vi "Main.vi"() -> ()   [LabVIEW 2012]
doc: "该连续测量范例项目在队列消息处理器模板的基础上实现。\n\n事件处理循环负责按用户界面操作生成对应的消息。\n\n消息处理循环负责对事件处理循环或其他消息生成的消息进行处理。其中还包括用于采集和记录消息处理循环的子VI，以及用于更新图表的循环。"
uses:
  Settings/Settings.ctl
  Acquisition/Hardware Configuration.ctl
  Acquisition/Signal Type.ctl
  Logging/Logging Configuration.ctl
  controls/UI Data.ctl
  Acquisition/Acquisition.lvlib
  Logging/Logging.lvlib
  Settings/Settings.lvlib
  support/User Event - Stop/User Event - Stop.lvlib
  support/Message Queue/Message Queue.lvlib
  Testing/Testing.lvlib
panel:
  out "数据":waveform(dbl)[](graph)
  in  "空白按钮 6":bool
  in  "?":bool
  in  "风机测试":bool
  in  "滚刷测试":bool
  in  "边刷测试":bool
  in  "行走轮测试":bool
  in  "设置":bool
  in  "整机测试开始":bool
  in  "停止":bool
  out "状态":string
  in  "紧急停止按钮":bool
  in  "退出":bool
  # "连续测量数据记录器"
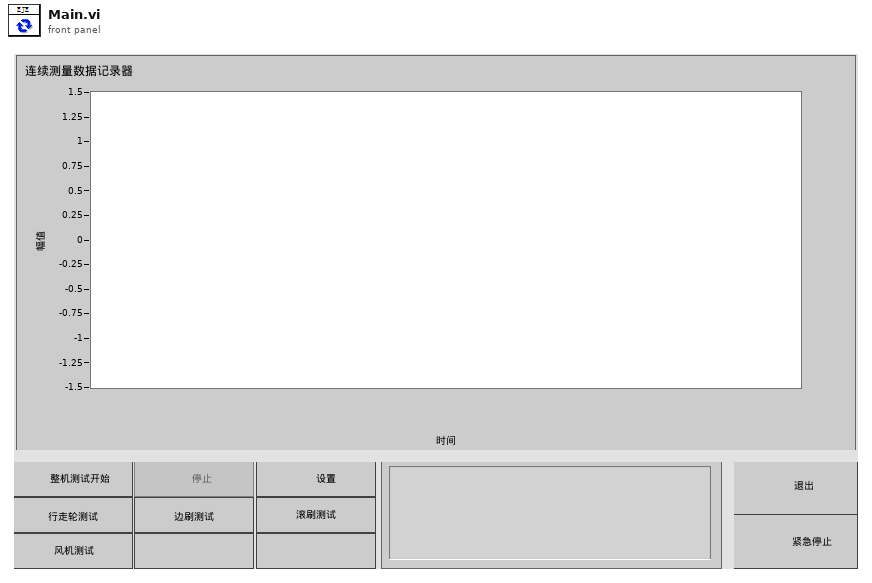
[diagram p1: front panel]
types:
  T1 = typedef "UI Data.ctl" = cluster{"开始引用":refnum<vi>, "停止引用":refnum<vi>, "设置引用":refnum<vi>, "退出引用":refnum<vi>, "状态引用":refnum<vi>, "数据引用":refnum<vi>}
  T2 = typedef "Settings.lvlib/Settings.ctl" = cluster{"硬件配置":T3, "记录配置":T5}
  T3 = typedef "Acquisition.lvlib/Hardware Configuration.ctl" = cluster{"硬件引用句柄<替换此项>":string, "信号类型<替换该项>":T4, "VISA资源名称":refnum<visa-resource-name>}
  T4 = typedef "Acquisition.lvlib/Signal Type.ctl" = enum16{"Sine Wave", "Square with Noise"}
  T5 = typedef "Logging.lvlib/Logging Configuration.ctl" = cluster{"记录文件基路径":path, "TDMS文件引用":refnum<k34>}
  T6 = typedef "Message Queue.lvlib/All Message Queues.ctl" = cluster{"UI":refnum<queue>, "采集":refnum<queue>, "记录":refnum<queue>}
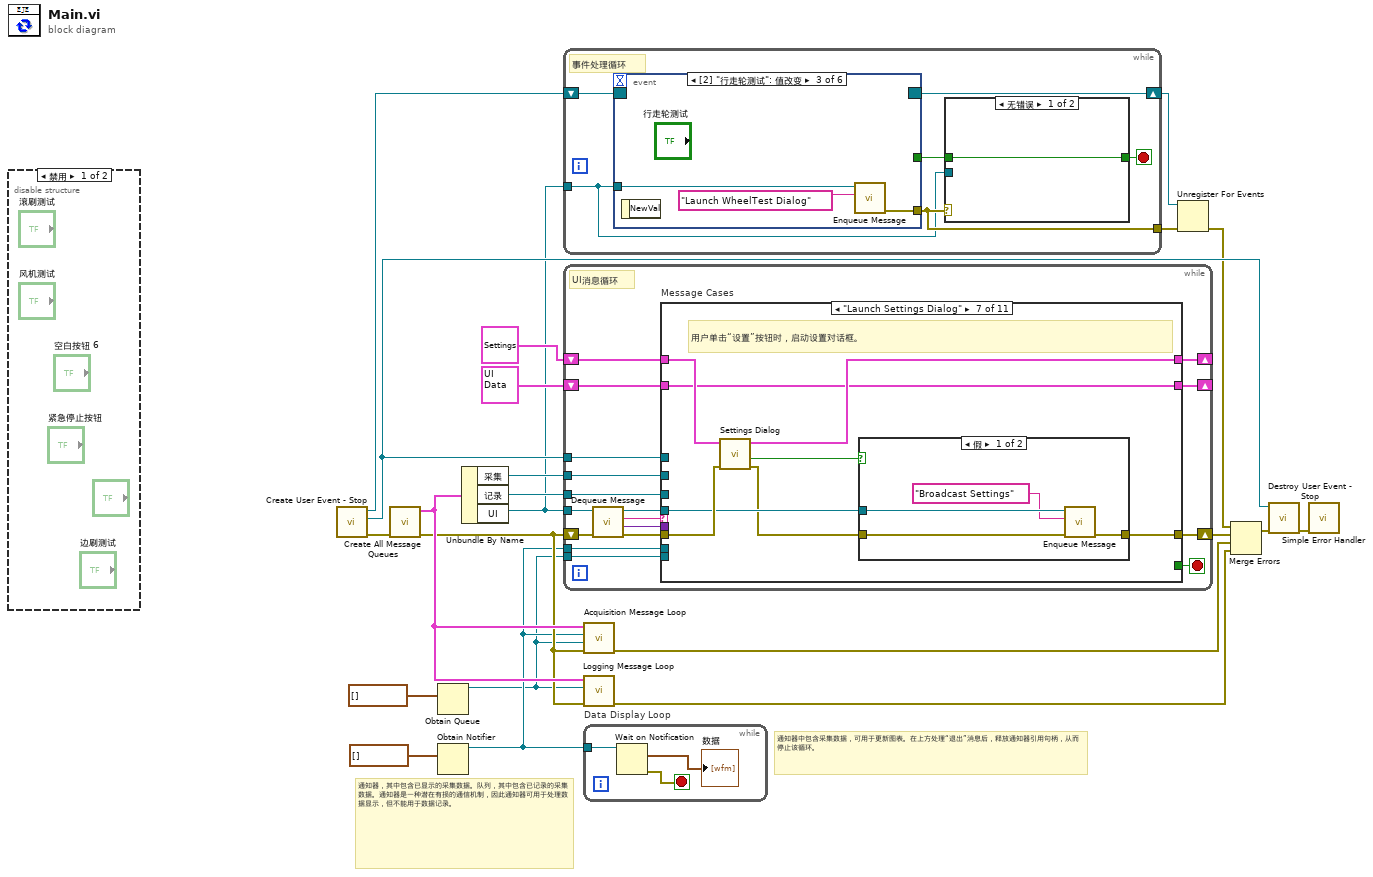
[diagram p0: block diagram]
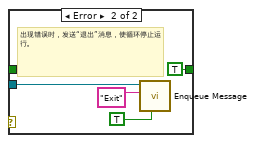
[diagram p3: hidden frame]
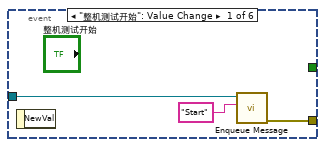
[diagram p4: hidden frame]
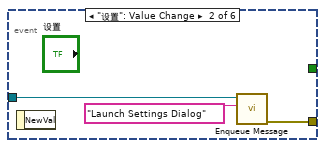
[diagram p5: hidden frame]
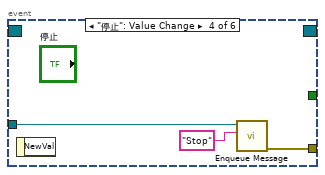
[diagram p6: hidden frame]
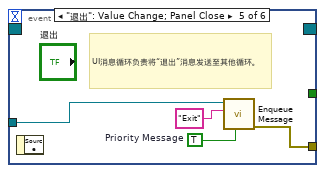
[diagram p7: hidden frame]
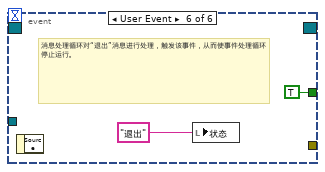
[diagram p8: hidden frame]
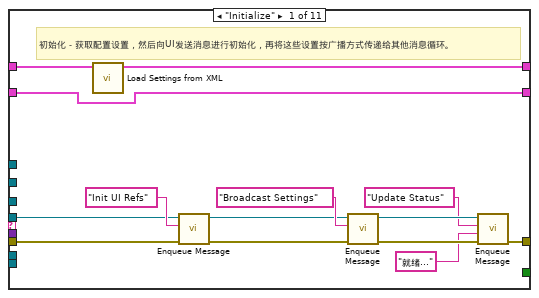
[diagram p9: hidden frame]
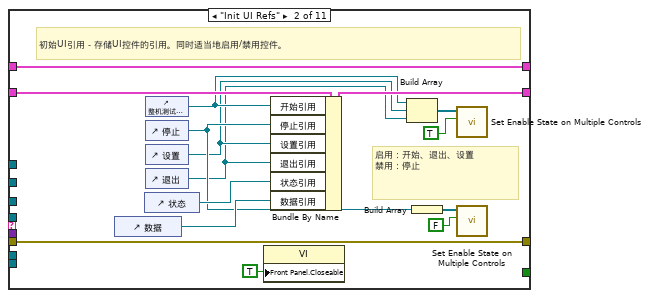
[diagram p10: hidden frame]
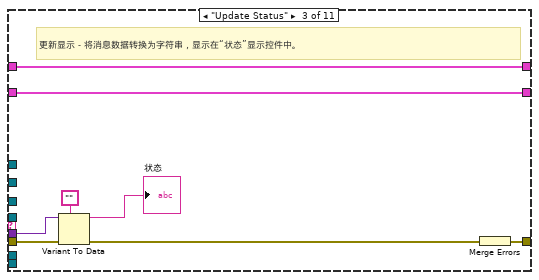
[diagram p11: hidden frame]
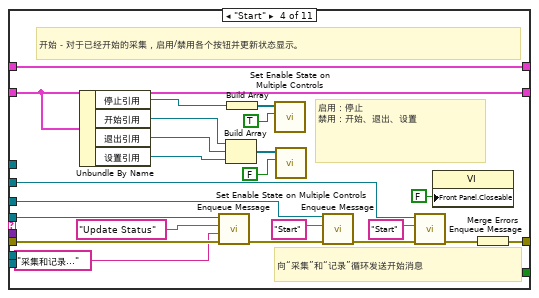
[diagram p12: hidden frame]
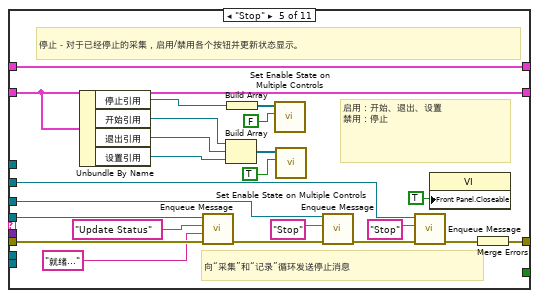
[diagram p13: hidden frame]
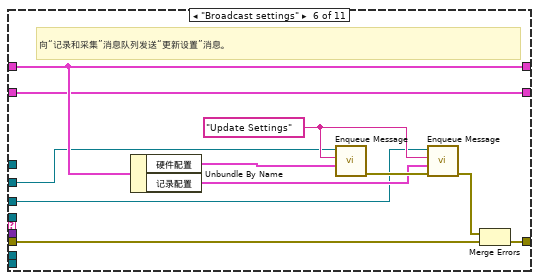
[diagram p14: hidden frame]
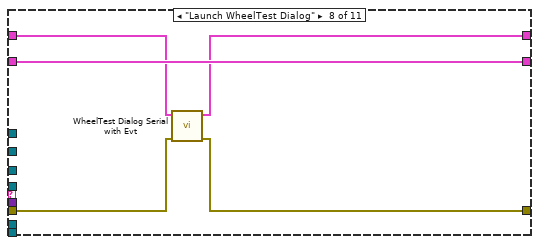
[diagram p16: hidden frame]
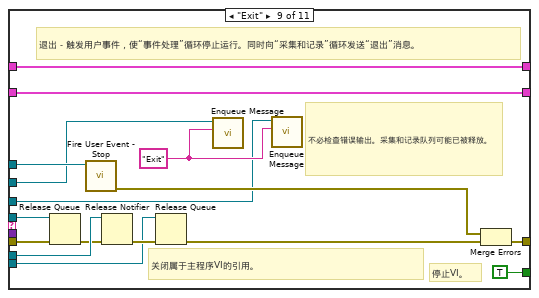
[diagram p17: hidden frame]
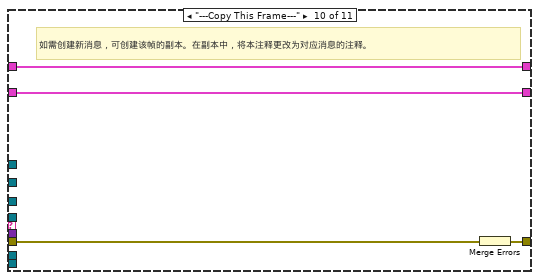
[diagram p18: hidden frame]
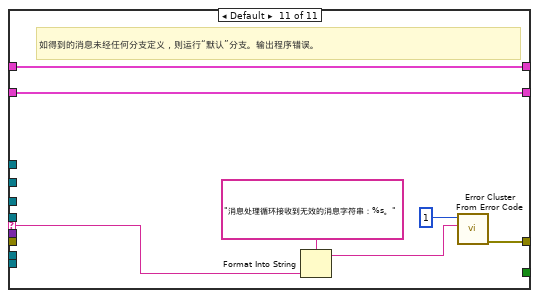
[diagram p19: hidden frame]
diagram:
  # "通知器，其中包含已显示的采集数据。队列，其中包含已记录的采集数据。通知器是一种潜在有损的通信机制，因此通知器可用于处理数据显示，但不能用于数据记录。"
  # "通知器中包含采集数据，可用于更新图表。在上方处理“退出”消息后，释放通知器引用句柄，从而停止该循环。"
  n1 = disable-structure shown="禁用" {
    frame Disabled {
    }
    frame Enabled {
    }
  }
  n2 = call "Create User Event - Stop.vi"() -> ("error out"=w16:cluster{"状态":bool, "代码":i32, "源":string}, "用户事件－停止"=w18:refnum<user-event>, "停止事件注册引用句柄"=w19:refnum<event-registration>)  [unwired: 9 in]
  n3 = call "Create All Message Queues.vi"("error in (no error)"=w16) -> ("error out"=w13:cluster{"状态":bool, "代码":i32, "源":string}, "消息队列输出"=w15:T6)  [unwired: 9 in]
  n4 = Obtain Queue(element data type=waveform(dbl)[] []) -> (queue out=w1:refnum<queue>)  [unwired: 4 in, 2 out]
  n5 = Obtain Notifier(notification data type=waveform(dbl)[] []) -> (notifier out=w3:refnum<notifier>)  [unwired: 3 in, 2 out]
  n6 = Unbundle By Name(w15) -> ("采集"=w8:refnum<queue>, "记录"=w7:refnum<queue>, "UI"=w6:refnum<queue>)
  n7 = while {
    tunnel: w6 -> [w24]
    tunnel: [w26] -> w21
    shift-right: [w23] -> w10
    shift-left: w19 -> [w25]
    stop <- w27 stop-if-true
    # "事件处理循环"
    n8 = event shown="[2] \"行走轮测试\": 值改变" {
      selector: w25 -> [_ _ _ _ _ _]
      dyn-events: [_ _ _ _ _ _] -> w23
      timeout: _ -> [_ _ _ _ _ _]
      tunnel: [_ _ _ _ _ TRUE ("Discard?")] -> w28
      tunnel: w24 -> [w34 w37 w41 w44 w46 _]
      tunnel: [w36 w39 w40 w43 w49 _] -> w26
      event "整机测试开始": Value Change {
        n9 = event-data() -> ()  [unwired: 1 in, 1 out]
        n10 = call "Enqueue Message.vi"("消息"="Start" ("Message"), "消息队列"=w34) -> ("error out"=w36:cluster{"状态":bool, "代码":i32, "源":string})  [unwired: 8 in, 1 out]
      }
      event "设置": Value Change {
        n11 = event-data() -> ()  [unwired: 1 in, 1 out]
        n12 = call "Enqueue Message.vi"("消息"="Launch Settings Dialog" ("Message"), "消息队列"=w37) -> ("error out"=w39:cluster{"状态":bool, "代码":i32, "源":string})  [unwired: 8 in, 1 out]
      }
      event "行走轮测试": Value Change {
        n13 = event-data() -> ()  [unwired: 1 in, 1 out]
        n14 = call "Enqueue Message.vi"("消息"="Launch WheelTest Dialog" ("Message"), "消息队列"=w41) -> ("error out"=w40:cluster{"状态":bool, "代码":i32, "源":string})  [unwired: 8 in, 1 out]
      }
      event "停止": Value Change {
        n15 = event-data() -> ()  [unwired: 1 in, 1 out]
        n16 = call "Enqueue Message.vi"("消息"="Stop" ("Message"), "消息队列"=w44) -> ("error out"=w43:cluster{"状态":bool, "代码":i32, "源":string})  [unwired: 8 in, 1 out]
      }
      event "退出": Value Change; Panel Close {
        w47 = TRUE  # Priority Message
        # "UI消息循环负责将“退出”消息发送至其他循环。"
        n17 = event-data() -> ()  [unwired: 1 in, 1 out]
        n18 = call "Enqueue Message.vi"("优先消息？(F)"=w47, "消息"="Exit" ("Message"), "消息队列"=w46) -> ("error out"=w49:cluster{"状态":bool, "代码":i32, "源":string})  [unwired: 7 in, 1 out]
      }
      event User Event {
        # "消息处理循环对“退出”消息进行处理，触发该事件，从而使事件处理循环停止运行。"
        n19 = event-data() -> ()  [unwired: 1 in, 1 out]
        n20 = local write "状态"("退出" ("Exit String")) -> ()
      }
    }
    n21 = case shown="无错误" w26 {
      tunnel: [w29 TRUE ("Discard?")] -> w27
      tunnel: w28 -> [w29 _]
      tunnel: w24 -> [_ w30]
      frame No Error {
      }
      frame Error {
        # "出现错误时，发送“退出”消息，使循环停止运行。"
        n22 = call "Enqueue Message.vi"("优先消息？(F)"=TRUE ("Discard?"), "消息"="Exit" ("Message"), "消息队列"=w30) -> ()  [unwired: 7 in, 2 out]
      }
    }
  }
  n23 = while {
    tunnel: w6 -> [w60]
    tunnel: w18 -> [w66]
    shift-right: [w67] -> w22
    shift-left: w13 -> [w65]
    shift-right: [w59] -> _
    shift-left: T2 {"硬件配置"={"硬件引用句柄<替换此项>"="", "信号类型<替换该项>"=enum."Sine Wave", "VISA资源名称"=""}, "记录配置"={"记录文件基路径"=path "", "TDMS文件引用"=refnum}} ("Settings") -> [w58]
    shift-right: [w56] -> _
    shift-left: T1 {"开始引用"=refnum, "停止引用"=refnum, "设置引用"=refnum, "退出引用"=refnum, "状态引用"=refnum, "数据引用"=refnum} ("Measurement UI Controls") -> [w57]
    tunnel: w8 -> [w55]
    tunnel: w7 -> [w54]
    tunnel: w3 -> [w53]
    tunnel: w1 -> [w52]
    stop <- w68 stop-if-true
    # "UI消息循环"
    n24 = call "Dequeue Message.vi"("error in (no error)"=w65, "消息队列"=w60) -> ("error out"=w64:cluster{"状态":bool, "代码":i32, "源":string}, "消息数据"=w62:variant, "消息"=w63:string, "消息队列副本"=w61:refnum<queue>)  [unwired: 6 in]
    n25 = case "Message Cases" shown="\"Launch Settings Dialog\"" w63 {
      selector: w63 -> [_ _ _ _ _ _ _ _ _ _ w206]
      tunnel: w61 -> [w72 _ _ w127 w150 _ w167 _ w186 _ _]
      tunnel: w64 -> [w71 w97 w104 w126 w149 w156 w169 w177 w194 w200 _]
      tunnel: [w78 w97 w105 w128 w151 w162 w164 w176 w195 w199 w204] -> w67
      tunnel: [_ _ _ _ _ _ _ _ TRUE _ _] -> w68
      tunnel: w62 -> [_ _ w103 _ _ _ _ _ _ _ _]
      tunnel: w66 -> [_ _ _ _ _ _ _ _ w193 _ _]
      tunnel: [w81 w96 w99 w125 w148 w160 w166 w178 w191 w198 w202] -> w59
      tunnel: w58 -> [w82 w96 w99 w125 w148 w160 w170 w179 w191 w198 w202]
      tunnel: w57 -> [w74 w95 w98 w122 w145 w154 w163 w180 w189 w197 w201]
      tunnel: [w74 w92 w98 w122 w145 w154 w163 w180 w189 w197 w201] -> w56
      tunnel: w55 -> [_ _ _ w108 w131 w153 _ _ w188 _ _]
      tunnel: w54 -> [_ _ _ w111 w134 w152 _ _ w187 _ _]
      tunnel: w53 -> [_ _ _ _ _ _ _ _ w185 _ _]
      tunnel: w52 -> [_ _ _ _ _ _ _ _ w181 _ _]
      frame "Initialize" {
        # "初始化－获取配置设置，然后向UI发送消息进行初始化，再将这些设置按广播方式传递给其他消息循环。"
        n26 = call "Load Settings from XML.vi"("设置输入"=w82) -> ("设置输出"=w81:T2)  [unwired: 9 in, 1 out]
        n27 = call "Enqueue Message.vi"("error in (no error)"=w71, "消息"="Init UI Refs" ("Message"), "消息队列"=w72) -> ("error out"=w69:cluster{"状态":bool, "代码":i32, "源":string}, "消息队列副本"=w70:refnum<queue>)  [unwired: 7 in]
        n28 = call "Enqueue Message.vi"("error in (no error)"=w69, "消息"="Broadcast Settings" ("Message"), "消息队列"=w70) -> ("error out"=w80:cluster{"状态":bool, "代码":i32, "源":string}, "消息队列副本"=w79:refnum<queue>)  [unwired: 7 in]
        n29 = call "Enqueue Message.vi"("error in (no error)"=w80, "消息数据"="就绪..." ("Ready..."), "消息"="Update Status" ("Message"), "消息队列"=w79) -> ("error out"=w78:cluster{"状态":bool, "代码":i32, "源":string})  [unwired: 6 in, 1 out]
      }
      frame "Init UI Refs" {
        # "启用：开始、退出、设置\n禁用：停止"
        # "初始UI引用－存储UI控件的引用。同时适当地启用/禁用控件。"
        n30 = control-ref of="数据"() -> (w93:refnum<vi>)
        n31 = control-ref of="状态"() -> (w94:refnum<vi>)
        n32 = control-ref of="整机测试开始"() -> (w86:refnum<vi>)
        n33 = control-ref of="停止"() -> (w87:refnum<vi>)
        n34 = control-ref of="设置"() -> (w85:refnum<vi>)
        n35 = control-ref of="退出"() -> (w84:refnum<vi>)
        n36 = property class="VI"("Front Panel.Closeable"=TRUE ("Front Panel Window:Closeable")) -> ()  [unwired: 2 in, 2 out]
        n37 = Bundle By Name(cluster=w95, "开始引用"=w86, "停止引用"=w87, "设置引用"=w85, "退出引用"=w84, "状态引用"=w94, "数据引用"=w93) -> (w92:T1)
        n38 = Build Array(w86, w85, w84) -> (w90:refnum<vi>[])
        n39 = Build Array(w87) -> (w89:refnum<vi>[])
        n40 = call "Set Enable State on Multiple Controls.vi"("启用？"=TRUE ("Enable?"), "控件"=w90) -> ()  [unwired: 10 in]
        n41 = call "Set Enable State on Multiple Controls.vi"("启用？"=FALSE ("Enable?"), "控件"=w89) -> ()  [unwired: 10 in]
      }
      frame "Update Status" {
        # "更新显示－将消息数据转换为字符串，显示在“状态”显示控件中。"
        n42 = Variant To Data(error in=w104, type="", Variant=w103) -> (data=→"状态":string, error out=w101:errorcluster)
        n43 = Merge Errors(w101) -> (w105:errorcluster)
      }
      frame "Start" {
        # "向“采集”和“记录”循环发送开始消息"
        # "启用：停止\n禁用：开始、退出、设置"
        # "开始－对于已经开始的采集，启用/禁用各个按钮并更新状态显示。"
        n44 = Unbundle By Name(w122) -> ("停止引用"=w117:refnum<vi>, "开始引用"=w116:refnum<vi>, "退出引用"=w115:refnum<vi>, "设置引用"=w114:refnum<vi>)
        n45 = call "Enqueue Message.vi"("error in (no error)"=w126, "消息数据"="采集和记录..." ("Acquiring and Logging..."), "消息"="Update Status" ("Message"), "消息队列"=w127) -> ("error out"=w113:cluster{"状态":bool, "代码":i32, "源":string})  [unwired: 6 in, 1 out]
        n46 = Build Array(w116, w115, w114) -> (w120:refnum<vi>[])
        n47 = Build Array(w117) -> (w119:refnum<vi>[])
        n48 = call "Set Enable State on Multiple Controls.vi"("启用？"=TRUE ("Enable?"), "控件"=w119) -> ()  [unwired: 10 in]
        n49 = call "Set Enable State on Multiple Controls.vi"("启用？"=FALSE ("Enable?"), "控件"=w120) -> ()  [unwired: 10 in]
        n50 = call "Enqueue Message.vi"("error in (no error)"=w113, "消息"="Start" ("Message"), "消息队列"=w111) -> ("error out"=w110:cluster{"状态":bool, "代码":i32, "源":string})  [unwired: 7 in, 1 out]
        n51 = call "Enqueue Message.vi"("error in (no error)"=w110, "消息"="Start" ("Message"), "消息队列"=w108) -> ("error out"=w109:cluster{"状态":bool, "代码":i32, "源":string})  [unwired: 7 in, 1 out]
        n52 = property class="VI"("Front Panel.Closeable"=FALSE ("Front Panel Window:Closeable")) -> ()  [unwired: 2 in, 2 out]
        n53 = Merge Errors(w109) -> (w128:errorcluster)
      }
      frame "Stop" {
        # "向“采集”和“记录”循环发送停止消息"
        # "启用：开始、退出、设置\n禁用：停止"
        # "停止－对于已经停止的采集，启用/禁用各个按钮并更新状态显示。"
        n54 = Unbundle By Name(w145) -> ("停止引用"=w140:refnum<vi>, "开始引用"=w139:refnum<vi>, "退出引用"=w138:refnum<vi>, "设置引用"=w137:refnum<vi>)
        n55 = call "Enqueue Message.vi"("error in (no error)"=w149, "消息数据"="就绪..." ("Ready..."), "消息"="Update Status" ("Message"), "消息队列"=w150) -> ("error out"=w136:cluster{"状态":bool, "代码":i32, "源":string})  [unwired: 6 in, 1 out]
        n56 = Build Array(w139, w138, w137) -> (w143:refnum<vi>[])
        n57 = Build Array(w140) -> (w142:refnum<vi>[])
        n58 = call "Set Enable State on Multiple Controls.vi"("启用？"=FALSE ("Enable?"), "控件"=w142) -> ()  [unwired: 10 in]
        n59 = call "Set Enable State on Multiple Controls.vi"("启用？"=TRUE ("Enable?"), "控件"=w143) -> ()  [unwired: 10 in]
        n60 = call "Enqueue Message.vi"("error in (no error)"=w136, "消息"="Stop" ("Message"), "消息队列"=w134) -> ("error out"=w133:cluster{"状态":bool, "代码":i32, "源":string})  [unwired: 7 in, 1 out]
        n61 = call "Enqueue Message.vi"("error in (no error)"=w133, "消息"="Stop" ("Message"), "消息队列"=w131) -> ("error out"=w132:cluster{"状态":bool, "代码":i32, "源":string})  [unwired: 7 in, 1 out]
        n62 = property class="VI"("Front Panel.Closeable"=TRUE ("Front Panel Window:Closeable")) -> ()  [unwired: 2 in, 2 out]
        n63 = Merge Errors(w132) -> (w151:errorcluster)
      }
      frame "Broadcast settings" {
        w155 = "Update Settings" ("Message")
        # "向“记录和采集”消息队列发送“更新设置”消息。"
        n64 = Unbundle By Name(w160) -> ("硬件配置"=w159:T3, "记录配置"=w158:T5)
        n65 = call "Enqueue Message.vi"("消息数据"=w159, "消息"=w155, "消息队列"=w153) -> ("error out"=w161:cluster{"状态":bool, "代码":i32, "源":string})  [unwired: 7 in, 1 out]
        n66 = call "Enqueue Message.vi"("error in (no error)"=w161, "消息数据"=w158, "消息"=w155, "消息队列"=w152) -> ("error out"=w157:cluster{"状态":bool, "代码":i32, "源":string})  [unwired: 6 in, 1 out]
        n67 = Merge Errors(w157, w156) -> (w162:errorcluster)
      }
      frame "Launch Settings Dialog" {
        # "用户单击“设置”按钮时，启动设置对话框。"
        n68 = call "Settings Dialog.vi"("error in (no error)"=w169, "设置输入"=w170) -> ("error out"=w165:cluster{"状态":bool, "代码":i32, "源":string}, "取消？"=w168:bool, "设置输出"=w166:T2)  [unwired: 6 in, 1 out]
        n69 = case shown="假" w168 {
          tunnel: w167 -> [w174 _]
          tunnel: w165 -> [w173 w175]
          tunnel: [w172 w175] -> w164
          frame False {
            n70 = call "Enqueue Message.vi"("error in (no error)"=w173, "消息"="Broadcast Settings" ("Message"), "消息队列"=w174) -> ("error out"=w172:cluster{"状态":bool, "代码":i32, "源":string})  [unwired: 7 in, 1 out]
          }
          frame True {
          }
        }
      }
      frame "Launch WheelTest Dialog" {
        n71 = call "WheelTest Dialog Serial with Evt.vi"("error in (no error)"=w177, "设置输入"=w179) -> ("error in (no error) 2"=w176:cluster{"状态":bool, "代码":i32, "源":string}, "设置输出"=w178:T2)  [unwired: 8 in]
      }
      frame "Exit" {
        w190 = "Exit" ("Message")
        # "不必检查错误输出。采集和记录队列可能已被释放。"
        # "关闭属于主程序VI的引用。"
        # "停止VI。"
        # "退出－触发用户事件，使“事件处理”循环停止运行。同时向“采集和记录”循环发送“退出”消息。"
        n72 = Release Queue(queue=w186, error in (no error)=w194) -> (error out=w184:errorcluster)  [unwired: 1 in, 2 out]
        n73 = call "Fire User Event - Stop.vi"("用户事件－停止"=w193) -> ("error out"=w192:cluster{"状态":bool, "代码":i32, "源":string})  [unwired: 10 in]
        n74 = Release Notifier(notifier=w185, error in (no error)=w184) -> (error out=w183:errorcluster)  [unwired: 1 in, 2 out]
        n75 = Release Queue(queue=w181, error in (no error)=w183) -> (error out=w182:errorcluster)  [unwired: 1 in, 2 out]
        n76 = call "Enqueue Message.vi"("消息"=w190, "消息队列"=w188) -> ()  [unwired: 8 in, 2 out]
        n77 = call "Enqueue Message.vi"("消息"=w190, "消息队列"=w187) -> ()  [unwired: 8 in, 2 out]
        n78 = Merge Errors(w192, w182) -> (w195:errorcluster)
      }
      frame "---Copy This Frame---" {
        # "如需创建新消息，可创建该帧的副本。在副本中，将本注释更改为对应消息的注释。"
        n79 = Merge Errors(w200) -> (w199:errorcluster)
      }
      frame Default {
        # "如得到的消息未经任何分支定义，则运行“默认”分支。输出程序错误。"
        n80 = Format Into String(format string="消息处理循环接收到无效的消息字符串：%s。" ("Invalid Message Loop Message"), w206) -> (resulting string=w203:string)  [unwired: 2 in, 1 out]
        n81 = call <vilib>:"Error Cluster From Error Code.vi"("error message (\"\")"=w203, "error code (0)"=1) -> ("error out"=w204:errorcluster)  [unwired: 7 in]
      }
    }
  }
  n82 = call "Acquisition Message Loop.vi"("error in (no error)"=w13, "数据队列"=w1, "数据通知器"=w3, "消息队列"=w15) -> ("error out"=w17:cluster{"状态":bool, "代码":i32, "源":string})  [unwired: 7 in]
  n83 = call "Logging Message Loop.vi"("error in (no error)"=w13, "数据队列"=w1, "消息队列"=w15) -> ("error out"=w14:cluster{"状态":bool, "代码":i32, "源":string})  [unwired: 8 in]
  n84 = while "Data Display Loop" {
    tunnel: w3 -> [w210]
    stop <- w208 stop-if-true
    n85 = Wait on Notification(notifier=w210) -> (notification=→"数据":waveform(dbl)[], error out=w208:errorcluster)  [unwired: 3 in, 2 out]
  }
  n86 = Unregister For Events(event registration refnum=w10, error in=w21) -> (error out=w11:errorcluster)
  n87 = Merge Errors(w11, w22, w17, w14) -> (w20:errorcluster)
  n88 = call "Destroy User Event - Stop.vi"("error in (no error)"=w20, "用户事件－停止"=w18) -> ("error out"=w4:cluster{"状态":bool, "代码":i32, "源":string})  [unwired: 9 in]
  n89 = call <vilib>:"Simple Error Handler.vi"("error in (no error)"=w4) -> ()  [unwired: 4 in, 5 out]
